vi "SEPSIS.vi"() -> ()   [LabVIEW 2023]
panel:
  out "Sweaty skin":bool
  out "High heart Rate":bool
  out "Extreme body pain":bool
  out "Short of Breathe":bool
  out "Confusion":bool
  out "Fever":bool
  out "Description Box":string
  in  "Tab Control":T1(tab)
  in  "Sensor Data":T2 {"BP" scale=0.0..120.0; "SpO2" scale=0.0..120.0; "Heart Rate" scale=0.0..120.0; "Temperature" scale=0.0..110.0; "MAP" scale=0.0..130.0; "Respiration rate" scale=0.0..120.0}
  out "ECG WAVEFORM":dbl(graph)
  out "HEART BEAT":dbl(graph)
  out "TEMPERATURE SENSOR":dbl(graph)
  in  "Select sensor":T3(ring)
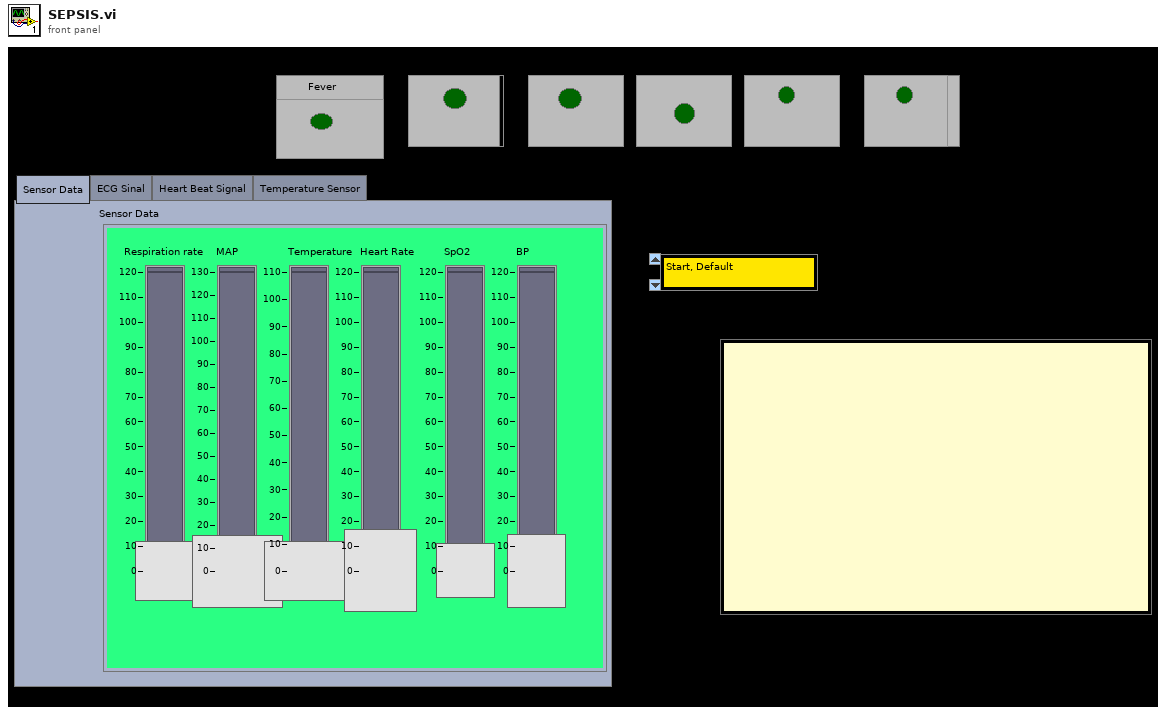
[diagram p1: front panel]
types:
  T1 = enum32{"Sensor Data", "ECG Sinal", "Heart Beat Signal", "Temperature Sensor"}
  T2 = cluster{"Respiration rate":dbl, "MAP":dbl, "Temperature":dbl, "Heart Rate":dbl, "SpO2":dbl, "BP":dbl}
  T3 = enum16{"Start, Default", "All Test", "Respiration", "MAP", "Temperature", "BP", "SpO2", "Heart Rate", "ECG Signal", "Temperature Sensor", "Heart Rate - Sensor", "Stop"}
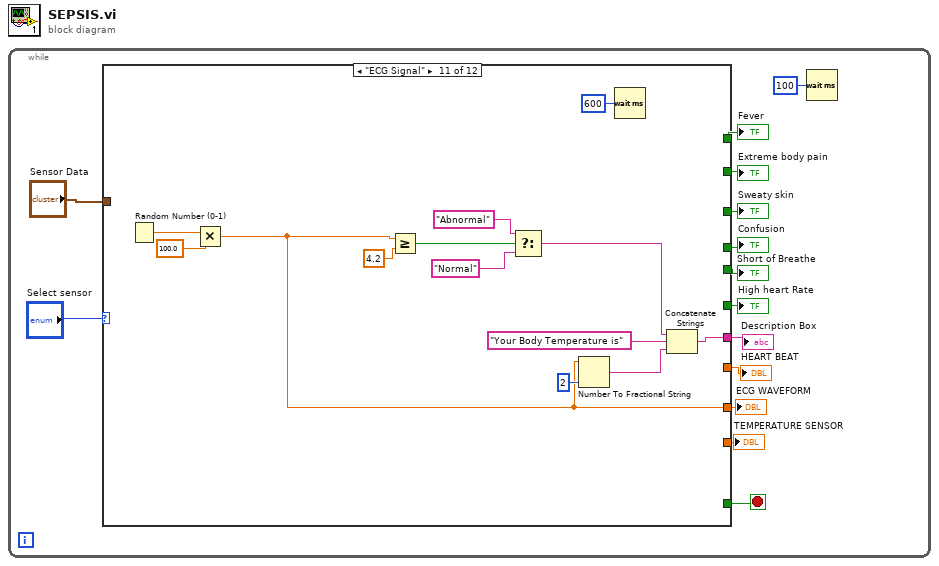
[diagram p0: block diagram]
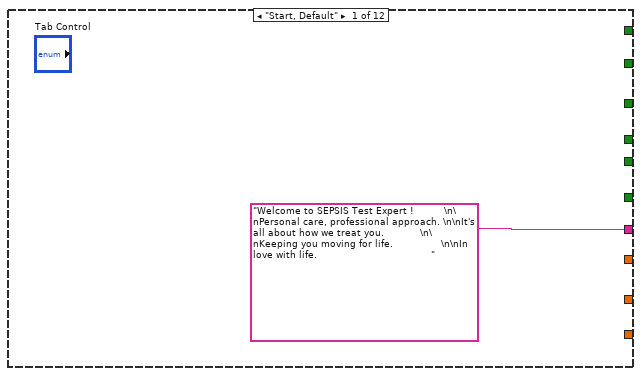
[diagram p2: hidden frame]
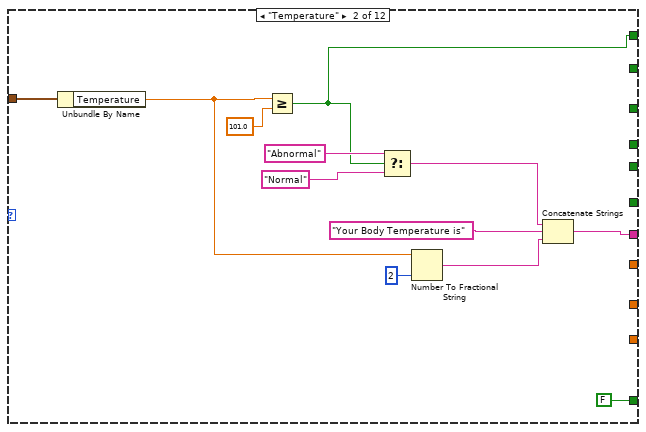
[diagram p3: hidden frame]
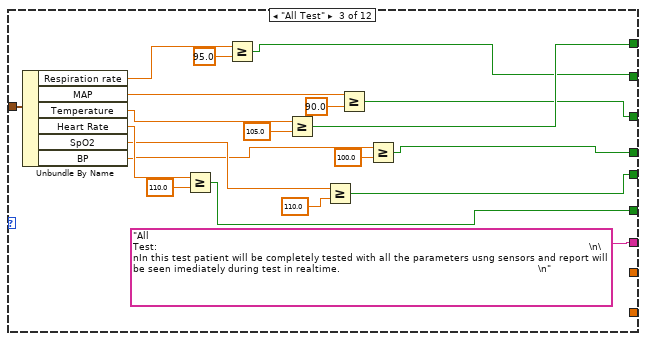
[diagram p4: hidden frame]
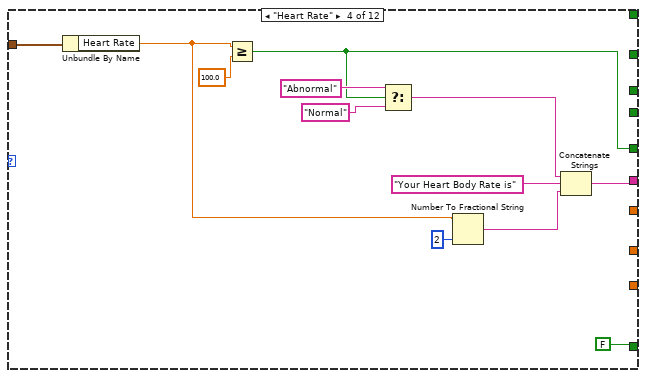
[diagram p5: hidden frame]
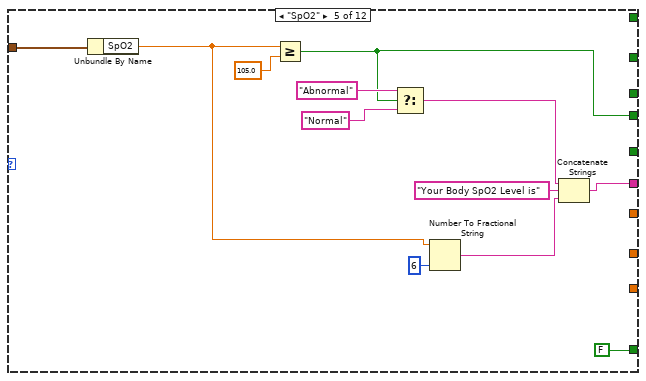
[diagram p6: hidden frame]
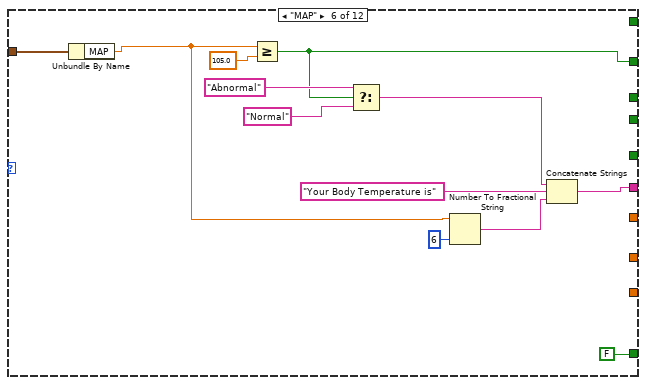
[diagram p7: hidden frame]
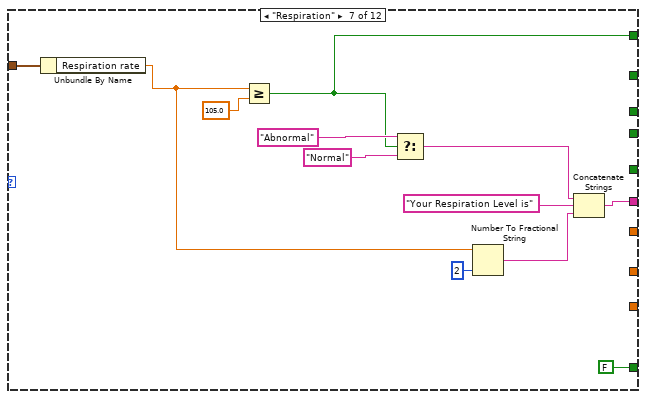
[diagram p8: hidden frame]
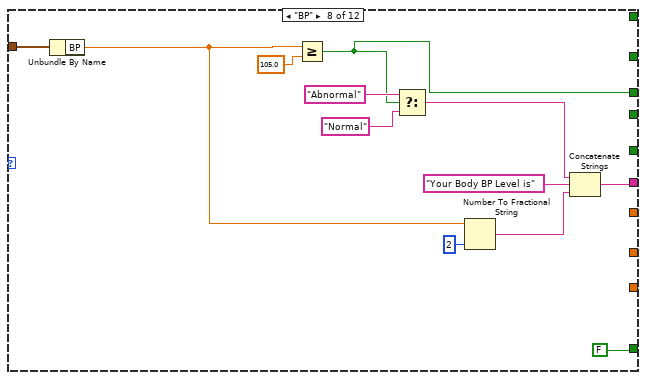
[diagram p9: hidden frame]
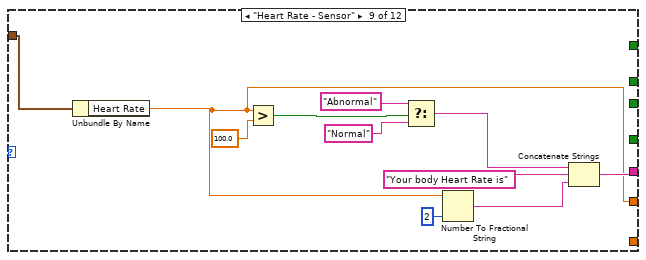
[diagram p10: hidden frame]
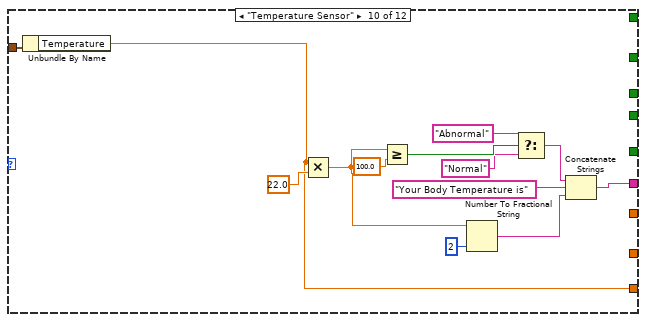
[diagram p11: hidden frame]
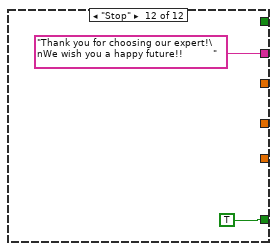
[diagram p12: hidden frame]
diagram:
  n1 = while {
    stop <- w11 stop-if-true
    n2 = case shown="\"ECG Signal\"" "Select sensor" {
      tunnel: "Sensor Data" -> [_ w27 w47 w59 w71 w82 w95 w107 w109 w120 _ _]
      tunnel: [_ w18 w33 _ _ _ _ _ _ _ _ _] -> w6
      tunnel: [_ _ w32 _ _ _ w86 _ _ _ _ _] -> w3
      tunnel: [_ _ w28 _ _ w75 _ _ _ _ _ _] -> w1
      tunnel: [_ _ w31 _ _ _ _ w98 _ _ _ _] -> w5
      tunnel: [_ _ w29 _ w62 _ _ _ _ _ _ _] -> w4
      tunnel: [_ _ w30 w54 _ _ _ _ _ _ _ _] -> w2
      tunnel: ["Welcome to SEPSIS Test Expert !          \n\nPersonal care, professional approach. \n\nIt's all about how we treat you.            \n\nKeeping you moving for life.                \n\nIn love with life.                                      " ("Description Box") w26 "All Test:                                                                                                                                                \n\nIn this test patient will be completely tested with all the parameters usng sensors and report will be seen imediately during test in realtime.                                                                  \n" ("Description Box") w48 w60 w83 w94 w103 w118 w131 w144 "Thank you for choosing our expert!\nWe wish you a happy future!!          " ("Description Box")] -> w12
      tunnel: [_ FALSE _ FALSE FALSE FALSE FALSE FALSE _ _ _ TRUE] -> w11
      tunnel: [_ _ _ _ _ _ _ _ _ w119 _ _] -> w10
      tunnel: [_ _ _ _ _ _ _ _ _ _ w133 _] -> w9
      tunnel: [_ _ _ _ _ _ _ _ w108 _ _ _] -> w8
      frame "Start, Default" {
      }
      frame "Temperature" {
        n3 = Unbundle By Name(w27) -> ("Temperature"=w17:dbl)
        n4 = Greater Or Equal?(x=w17, y=101.0) -> (x >= y?=w18:bool)
        n5 = Select(t="Abnormal", s=w18, f="Normal") -> (s? t:f=w20:string)
        n6 = Number To Fractional String(number=w17, precision (6)=i16 2) -> (F-format string=w24:string)  [unwired: 2 in]
        n7 = Concatenate Strings(w20, "Your Body Temperature is" ("string"), w24) -> (w26:string)
      }
      frame "All Test" {
        n8 = Unbundle By Name(w47) -> ("Respiration rate"=w46:dbl, "MAP"=w45:dbl, "Temperature"=w44:dbl, "Heart Rate"=w43:dbl, "SpO2"=w42:dbl, "BP"=w41:dbl)
        n9 = Greater Or Equal?(x=w43, y=110.0) -> (x >= y?=w30:bool)
        n10 = Greater Or Equal?(x=w46, y=95.0) -> (x >= y?=w32:bool)
        n11 = Greater Or Equal?(x=w44, y=105.0) -> (x >= y?=w33:bool)
        n12 = Greater Or Equal?(x=w42, y=110.0) -> (x >= y?=w29:bool)
        n13 = Greater Or Equal?(x=w45, y=90.0) -> (x >= y?=w28:bool)
        n14 = Greater Or Equal?(x=w41, y=100.0) -> (x >= y?=w31:bool)
      }
      frame "Heart Rate" {
        n15 = Unbundle By Name(w59) -> ("Heart Rate"=w49:dbl)
        n16 = Greater Or Equal?(x=w49, y=100.0) -> (x >= y?=w54:bool)
        n17 = Select(t="Abnormal", s=w54, f="Normal") -> (s? t:f=w52:string)
        n18 = Number To Fractional String(number=w49, precision (6)=i16 2) -> (F-format string=w57:string)  [unwired: 2 in]
        n19 = Concatenate Strings(w52, "Your Heart Body Rate is" ("string"), w57) -> (w48:string)
      }
      frame "SpO2" {
        n20 = Unbundle By Name(w71) -> ("SpO2"=w61:dbl)
        n21 = Greater Or Equal?(x=w61, y=105.0) -> (x >= y?=w62:bool)
        n22 = Select(t="Abnormal", s=w62, f="Normal") -> (s? t:f=w66:string)
        n23 = Number To Fractional String(number=w61, precision (6)=i16 6) -> (F-format string=w69:string)  [unwired: 2 in]
        n24 = Concatenate Strings(w66, "Your Body SpO2 Level is" ("string"), w69) -> (w60:string)
      }
      frame "MAP" {
        n25 = Unbundle By Name(w82) -> ("MAP"=w73:dbl)
        n26 = Greater Or Equal?(x=w73, y=105.0) -> (x >= y?=w75:bool)
        n27 = Select(t="Abnormal", s=w75, f="Normal") -> (s? t:f=w77:string)
        n28 = Number To Fractional String(number=w73, precision (6)=i16 6) -> (F-format string=w78:string)  [unwired: 2 in]
        n29 = Concatenate Strings(w77, "Your Body Temperature is" ("string"), w78) -> (w83:string)
      }
      frame "Respiration" {
        n30 = Unbundle By Name(w95) -> ("Respiration rate"=w85:dbl)
        n31 = Greater Or Equal?(x=w85, y=105.0) -> (x >= y?=w86:bool)
        n32 = Select(t="Abnormal", s=w86, f="Normal") -> (s? t:f=w88:string)
        n33 = Number To Fractional String(number=w85, precision (6)=i16 2) -> (F-format string=w89:string)  [unwired: 2 in]
        n34 = Concatenate Strings(w88, "Your Respiration Level is" ("string"), w89) -> (w94:string)
      }
      frame "BP" {
        n35 = Unbundle By Name(w107) -> ("BP"=w96:dbl)
        n36 = Greater Or Equal?(x=w96, y=105.0) -> (x >= y?=w98:bool)
        n37 = Select(t="Abnormal", s=w98, f="Normal") -> (s? t:f=w100:string)
        n38 = Number To Fractional String(number=w96, precision (6)=i16 2) -> (F-format string=w102:string)  [unwired: 2 in]
        n39 = Concatenate Strings(w100, "Your Body BP Level is" ("string"), w102) -> (w103:string)
      }
      frame "Heart Rate - Sensor" {
        n40 = Unbundle By Name(w109) -> ("Heart Rate"=w108:dbl)
        n41 = Greater?(x=w108, y=100.0) -> (0:w116:bool)
        n42 = Select(t="Abnormal", s=w116, f="Normal") -> (s? t:f=w112:string)
        n43 = Number To Fractional String(number=w108, precision (6)=i16 2) -> (F-format string=w113:string)  [unwired: 2 in]
        n44 = Concatenate Strings(w112, "Your body Heart Rate is" ("string"), w113) -> (w118:string)
      }
      frame "Temperature Sensor" {
        n45 = Unbundle By Name(w120) -> ("Temperature"=w119:dbl)
        n46 = Multiply(x=w119, y=22.0) -> (x*y=w123:dbl)
        n47 = Greater Or Equal?(x=w123, y=100.0) -> (x >= y?=w122:bool)
        n48 = Number To Fractional String(number=w123, precision (6)=i16 2) -> (F-format string=w130:string)  [unwired: 2 in]
        n49 = Select(t="Abnormal", s=w122, f="Normal") -> (s? t:f=w127:string)
        n50 = Concatenate Strings(w127, "Your Body Temperature is" ("string"), w130) -> (w131:string)
      }
      frame "ECG Signal" {
        n51 = Random Number (0-1)() -> (number: 0 to 1=w135:dbl)
        n52 = Multiply(x=w135, y=100.0) -> (x*y=w133:dbl)
        n53 = Greater Or Equal?(x=w133, y=4.2) -> (x >= y?=w137:bool)
        n54 = Select(t="Abnormal", s=w137, f="Normal") -> (s? t:f=w138:string)
        n55 = Number To Fractional String(number=w133, precision (6)=i16 2) -> (F-format string=w140:string)  [unwired: 2 in]
        n56 = Wait (ms)(milliseconds to wait=u32 600) -> ()  [unwired: 1 out]
        n57 = Concatenate Strings(w138, "Your Body Temperature is" ("string"), w140) -> (w144:string)
      }
      frame "Stop" {
      }
    }
    "Description Box" <- w12
    "HEART BEAT" <- w8
    "ECG WAVEFORM" <- w9
    "TEMPERATURE SENSOR" <- w10
    "Fever" <- w6
    "Confusion" <- w5
    "Short of Breathe" <- w4
    "Extreme body pain" <- w3
    "High heart Rate" <- w2
    "Sweaty skin" <- w1
    n58 = Wait (ms)(milliseconds to wait=u32 100) -> ()  [unwired: 1 out]
  }
